vi "ziModGetByteArray.vi"(8 "Error In":errorcluster, 10 "ModResults":T2, 11 "ModHandle In":T6 {"ModHandle" format="0x%08x"; "Conn" format="0x%08x"}) -> (0 "Error Out":errorcluster, 2 "ByteArray":T1[](array[typedef]), 3 "ModHandle Out":T6 {"ModHandle" format="0x%08x"; "Conn" format="0x%08x"})   [LabVIEW 2015, in "Zurich Instruments LabOne.lvlib"]
doc: "Use this vi to get ByteArrayData from a ModResult returned from ziModGetNextNode.vi. \nIt returns an array of BytesArrays."
uses:
  Zurich Instruments LabOne.lvlib
  Data/ziTypeByteArray.ctl
  Zurich Instruments/LabOne/API/LabVIEW/Zurich Instruments LabOne/Private/ziLV64.framework
  Data/ziTypePollType.ctl
  ziTypeModHandle.ctl
  ziTypeModResults.ctl
  ziTypeModSWTriggerHeader.ctl
  ziTypeModSweeperHeader.ctl
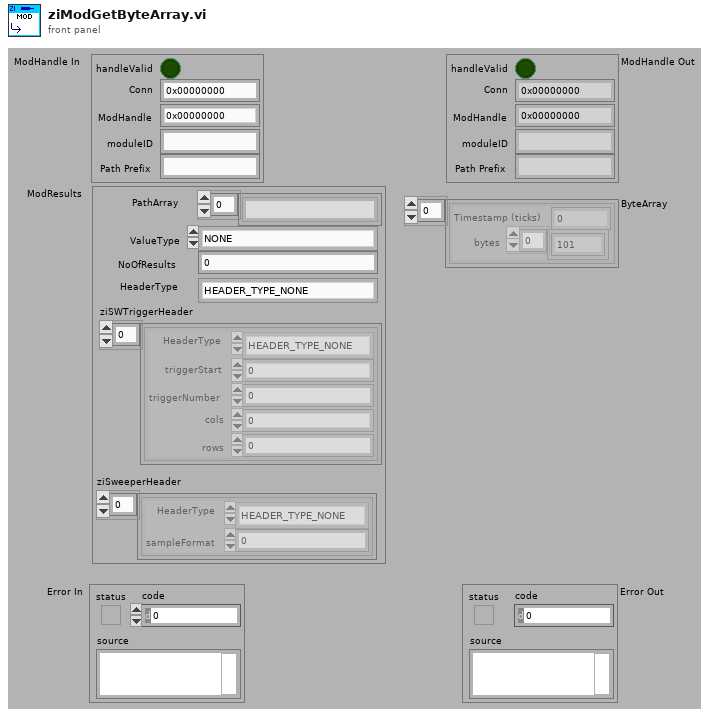
[diagram p1: front panel]
types:
  T1 = typedef "Zurich Instruments LabOne.lvlib/ziTypeByteArray.ctl" = cluster{"Timestamp (ticks)":u64, "bytes":i8[]}
  T2 = typedef "Zurich Instruments LabOne.lvlib/ziTypeModResults.ctl" = cluster{"PathArray":string[], "ValueType":T3, "NoOfResults":u64, "HeaderType":enum16{"HEADER_TYPE_NONE", "HEADER_TYPE_SWTRIGGER", "HEADER_TYPE_SWEEPER"}, "ziSWTriggerHeader":T4[], "ziSweeperHeader":T5[]}
  T3 = typedef "Zurich Instruments LabOne.lvlib/ziTypePollType.ctl" = enum16{"NONE", "DOUBLE_DATA", "INTEGER_DATA", "DEMOD_SAMPLE", "SCOPE_WAVE_HF2", "AUXIN_SAMPLE", "DIO_SAMPLE", "BYTE_ARRAY", "PWA_WAVE", "9", "10", "11", "12", "13", "14", "15", "TREE_CHANGE_DEPRI", "17", "ERROR", "19", "20", "21", "22", "23", "24", "25", "26", "27", "28", "29", "30", "31", "DOUBLE_DATA_TS", "INTEGER_DATA_TS", "34", "SCOPE_WAVE", "36", "37", "BYTE_ARRAY_TS", "39", "40", "41", "42", "43", "44", "45", "CNT_DATA", "47", "TREE_CHANGE", "49", "50", "51", "52", "53", "54", "55", "56", "57", "58", "59", "60", "61", "62", "63", "SWEEPER_DATA", "SPECTRUM_DATA", "ADVISOR_DATA", "67", "IMP_DATA"}
  T4 = typedef "Zurich Instruments LabOne.lvlib/ziTypeModSWTriggerHeader.ctl" = cluster{"HeaderType":enum8{"HEADER_TYPE_NONE", "HEADER_TYPE_SWTRIGGER", "HEADER_TYPE_SWEEPER"}, "triggerStart":u64, "triggerNumber":u64, "cols":u32, "rows":u32}
  T5 = typedef "Zurich Instruments LabOne.lvlib/ziTypeModSweeperHeader.ctl" = cluster{"HeaderType":enum8{"HEADER_TYPE_NONE", "HEADER_TYPE_SWTRIGGER", "HEADER_TYPE_SWEEPER"}, "sampleFormat":u8}
  T6 = typedef "Zurich Instruments LabOne.lvlib/ziTypeModHandle.ctl" = cluster{"handleValid":bool, "Conn":u64, "ModHandle":u64, "moduleID":string, "Path Prefix":string}
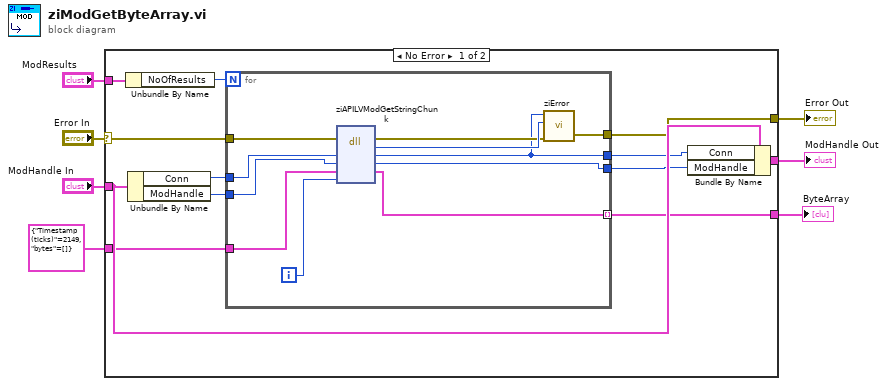
[diagram p0: block diagram]
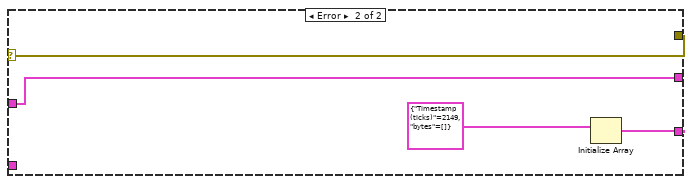
[diagram p2: hidden frame]
diagram:
  n1 = case shown="No Error" "Error In" {
    selector: "Error In" -> [w10 w33]
    tunnel: [w11 w33] -> w3
    tunnel: [w18 w34] -> w6
    tunnel: "ModHandle In" -> [w19 w34]
    tunnel: "ModResults" -> [w15 _]
    tunnel: [w8 w32] -> w1
    tunnel: T1 {"Timestamp (ticks)"=2149, "bytes"=[]} ("ByteArray") -> [w9 _]
    frame No Error {
      n2 = Unbundle By Name(w15) -> ("NoOfResults"=w14:u64)
      n3 = Unbundle By Name(w19) -> ("Conn"=w17:u64, "ModHandle"=w16:u64)
      n4 = for {
        N: w14 -> [_]
        tunnel: [w20] -> w13
        tunnel: [w30] -> w12
        tunnel: w17 -> [w29]
        tunnel: w16 -> [w28]
        tunnel: [w26] -> w11
        tunnel: w10 -> [w23]
        tunnel: w9 -> [w22]
        tunnel: [w21] -> w8 mode=indexing
        i -> [w27]
        n5 = dll-call lib="Users/arkady/Desktop/ado/github/resonant_ultrasound_arxiv/maglab ultrasound -- arkady --arxiv/Zurich Instruments/LabOne/API/LabVIEW/Zurich Instruments LabOne/Private/ziLV*.*" fn="ziAPILVModGetStringChunk" label="ziAPILVModGetSweeperWaveChunk"(error in=w23, "Conn"=w29, "ModHandle"=w28, "ByteArray"=w22, "chunk_idx"=w27) -> (error out=w24:errorcluster, "return type"=w25:u32, "Conn"=w20:u64, "ModHandle"=w30:u64, "ByteArray"=w21:T1)  [unwired: 3 in, 1 out]
        n6 = call "ziError.vi"("Conn"=w20, "ziErrorCode"=w25, "Error In"=w24) -> ("Error Out"=w26:errorcluster)  [unwired: 2 in, 1 out]
      }
      n7 = Bundle By Name(cluster=w19, "Conn"=w13, "ModHandle"=w12) -> (w18:T6)
    }
    frame Error {
      n8 = Initialize Array(T1 {"Timestamp (ticks)"=2149, "bytes"=[]} ("ByteArray")) -> (w32:T1[])  [unwired: 1 in]
    }
  }
  "Error Out" <- w3
  "ModHandle Out" <- w6
  "ByteArray" <- w1
